vi "PH_Calorimeter_USB.PC Set Time Base Settings.vi"(0 "i ref in":refnum<vi>, 2 "Rate [Hz]":i32, 5 "error in (no error)":errorcluster) -> (14 "i ref out":refnum<vi>, 19 "error out":errorcluster)   [LabVIEW 2014, in "PH_Calorimeter_USB.lvlib"]
doc: "This is the Proc Case done in \"SetTimeBaseSettings\": the samples per channel are calculated from the Rate, the T 1/e constant and the Wait Time, written to own attributes and the related GUI element. Do not use the VI inside \"get Data to modify / save modified data\" loop."
uses:
  PH_Calorimeter_USB.lvlib
  PH_Calorimeter_USB.Time Base Settings.ctl
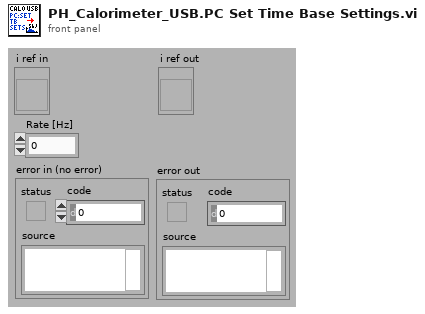
[diagram p1: front panel]
types:
  T1 = typedef "PH_Calorimeter_USB.lvlib/PH_Calorimeter_USB.i attribute.ctl" = cluster{"GUI Refs":cluster{"Delete":refnum<vi>, "Start":refnum<vi>, "Energy":refnum<vi>, "Calorimeter":refnum<vi>, "Trigger":refnum<vi>, "Calo Calibration":refnum<vi>, "Time Base":refnum<vi>, "Device":refnum<vi>, "Graph Raw Data":refnum<vi>, "Graph Result":refnum<vi>}, "DAQ Instance":string, "Data":dbl[][], "Controller Instance":string, "Energy [J]":dbl, "Calorimeter":T2, "Trigger":T3, "Time Base":T4, "Calo Calibration":T5, "Serial Number":string}
  T2 = typedef "PH_Calorimeter_USB.lvlib/PH_Calorimeter_USB.Calorimeter Settings.ctl" = cluster{"Channel":tag, "Min Value [V]":dbl, "Max Value  [V]":dbl}
  T3 = typedef "PH_Calorimeter_USB.lvlib/PH_Calorimeter_USB.Trigger Settings.ctl" = cluster{"Channel":tag, "Min Value [V]":dbl, "Max Value  [V]":dbl, "Level [V]":dbl, "Wait Time [s]":dbl, "Length [Samples]":i32}
  T4 = typedef "PH_Calorimeter_USB.lvlib/PH_Calorimeter_USB.Time Base Settings.ctl" = cluster{"Samples per Channel":i32, "Rate [Hz]":i32}
  T5 = typedef "PH_Calorimeter_USB.lvlib/PH_Calorimeter_USB.Calorimeter Calibration Settings.ctl" = cluster{"T 1/e [s]":dbl, "Sensitivity  [Vs/J]":dbl}
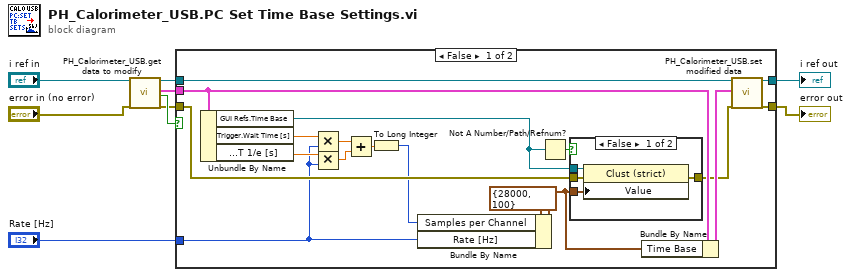
[diagram p0: block diagram]
diagram:
  n1 = call "PH_Calorimeter_USB.get data to modify.vi"("i ref in"="i ref in", "error in (no error)"="error in (no error)") -> ("i ref out"=w3:refnum<vi>, "i attribute"=w7:T1, "timed out"=w8:bool, "error out"=w5:errorcluster)  [unwired: 14 in]
  n2 = case shown="False" w8 {
    tunnel: w3 -> [w27 w34]
    tunnel: [w26 w34] -> w4
    tunnel: w5 -> [w21 w33]
    tunnel: [w25 w33] -> w6
    tunnel: w7 -> [w23 _]
    tunnel: "Rate [Hz]" -> [w11 _]
    frame False {
      n3 = Unbundle By Name(w23) -> ("GUI Refs.Time Base"=w12:refnum<vi>, "Trigger.Wait Time [s]"=w13:dbl, "Calo Calibration.T 1/e [s]"=w18:dbl)
      n4 = Multiply(x=w13, y=w11) -> (x*y=w16:dbl)
      n5 = Multiply(x=w18, y=w11) -> (x*y=w17:dbl)
      n6 = Add(x=w16, y=w17) -> (x+y=w19:dbl)
      n7 = To Long Integer(number=w19) -> (32bit integer=w10:i32)
      n8 = Bundle By Name(cluster=T4 {"Samples per Channel"=28000, "Rate [Hz]"=100} ("Time Base"), "Samples per Channel"=w10, "Rate [Hz]"=w11) -> (w14:T4)
      n9 = Not A Number/Path/Refnum?(number/path/refnum=w12) -> (NaN/Path/Refnum?=w22:bool)
      n10 = case shown="False" w22 {
        tunnel: w21 -> [w31 w32]
        tunnel: w12 -> [w30 _]
        tunnel: w14 -> [w29 _]
        tunnel: [w28 w32] -> w20
        frame False {
          n11 = property class="Clust (strict)"(reference=w30, error in=w31, "Value"=w29) -> (error out=w28:errorcluster)  [unwired: 1 out]
        }
        frame True {
        }
      }
      n12 = Bundle By Name(cluster=w23, "Time Base"=w14) -> (w24:T1)
      n13 = call "PH_Calorimeter_USB.set modified data.vi"("i ref in"=w27, "i attribute"=w24, "error in (no error)"=w20) -> ("i ref out"=w26:refnum<vi>, "error out"=w25:errorcluster)  [unwired: 15 in]
    }
    frame True {
    }
  }
  "error out" <- w6
  "i ref out" <- w4
